vi "PM100D_SYST-ERR.vi"(3 "error out 2":errorcluster, 5 "VISA In":refnum<visa-resource-name>) -> (0 "error out":errorcluster, 1 "Error":string, 2 "VISA Out":refnum<visa-resource-name>)   [LabVIEW 2014]
doc: "This VI lists all errors coming from the instrument\n'no error' is supressed"
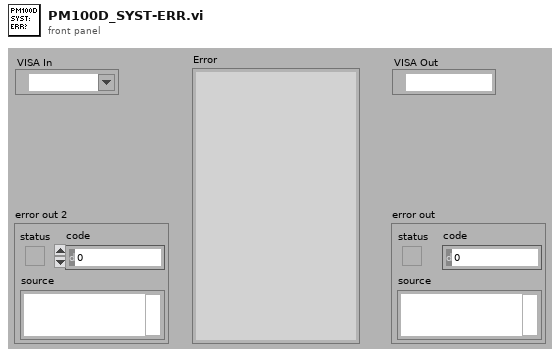
[diagram p1: front panel]
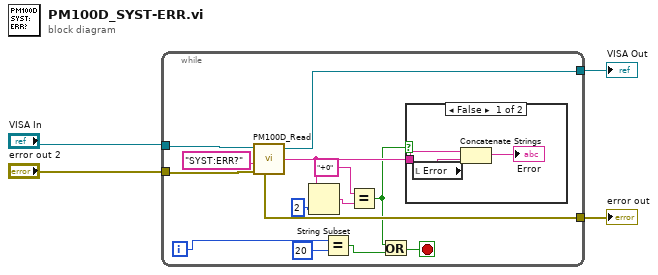
[diagram p0: block diagram]
diagram:
  n1 = while {
    tunnel: "VISA In" -> [w18]
    tunnel: "error out 2" -> [w17]
    tunnel: [w10] -> w3
    tunnel: [w9] -> w4
    i -> [w12]
    stop <- w14 stop-if-true
    n2 = call "PM100D_Read.vi"("error in (no error)"=w17, "Command"="SYST:ERR?", "VISA in"=w18) -> ("error out"=w9:errorcluster, "ReadValue"=w8:string, "VISA out"=w10:refnum<visa-resource-name>)  [unwired: 1 out]
    n3 = String Subset(string=w8, length (rest)=2 ("length (rest)")) -> (substring=w6:string)  [unwired: 1 out]
    n4 = Equal?(x=w12, y=20) -> (x = y?=w13:bool)
    n5 = Equal?(x="+0" ("y"), y=w6) -> (x = y?=w7:bool)
    n6 = Or(x=w7, y=w13) -> (x .or. y?=w14:bool)
    n7 = case shown="False" w7 {
      tunnel: w8 -> [w19 _]
      frame False {
        n8 = local read "Error"() -> (w20:string)
        n9 = Concatenate Strings(w19, w20) -> (→"Error":string)
      }
      frame True {
      }
    }
  }
  "error out" <- w4
  "VISA Out" <- w3
